vi "UDL-FileLibraryPath.vi"(8 "error in":errorcluster) -> (0 "error out":errorcluster, 3 "Library Filepath":path)   [LabVIEW 2013]
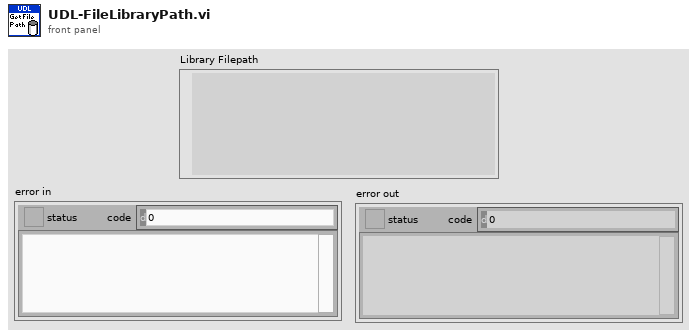
[diagram p1: front panel]
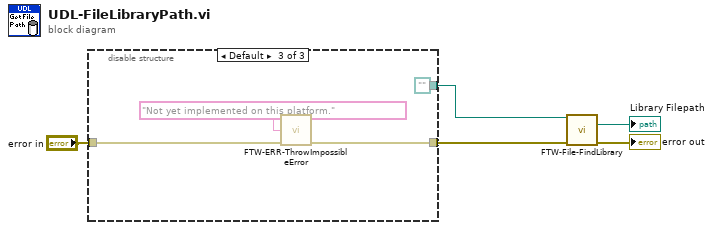
[diagram p0: block diagram]
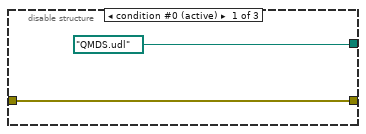
[diagram p2: hidden frame]
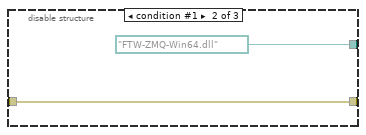
[diagram p3: hidden frame]
diagram:
  n1 = disable-structure shown="Default" {
    disable-tunnel: [path "QMDS.udl" path "FTW-ZMQ-Win64.dll" path ""] -> w4
    disable-tunnel: [w7 w9 w12] -> w3
    disable-tunnel: "error in" -> [w7 w9 w13]
    frame condition #0 (active) {
    }
    frame condition #1 {
    }
    frame condition #2 {
      n2 = call "FTW-ERR-ThrowImpossibleError.vi"("Reason this error should never happen"="Not yet implemented on this platform.", "error in"=w13) -> ("error out"=w12:errorcluster)  [unwired: 13 in]
    }
  }
  n3 = call "FTW-File-FindLibrary.vi"("Library File Pattern"=w4, "error in"=w3) -> ("Library Filepath"=→"Library Filepath":path, "error out"=→"error out":errorcluster)  [unwired: 12 in]
